vi "簇转换表格.vi"(11 "引用句柄":refnum<vi>) -> (3 "out":string[][](array[string]))   [LabVIEW 2018]
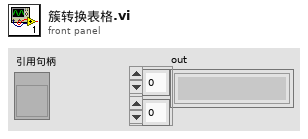
[diagram p1: front panel]
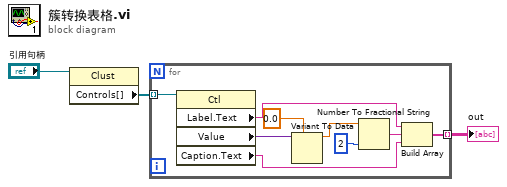
[diagram p0: block diagram]
diagram:
  n1 = property class="Clust"(reference="引用句柄") -> ("Controls[]"=w2:refnum<vi>[])  [unwired: 1 in, 2 out]
  n2 = for {
    tunnel: w2 -> [w10] mode=indexing
    tunnel: [w12] -> w3 mode=indexing
    n3 = property class="Ctl"(reference=w10) -> ("Label.Text"=w11:string, "Value"=w8:variant, "Caption.Text"=w9:string)  [unwired: 1 in, 2 out]
    n4 = Variant To Data(type=0.0, Variant=w8) -> (data=w5:dbl)  [unwired: 1 in, 1 out]
    n5 = Number To Fractional String(number=w5, precision (6)=i16 2 ("精度(6)")) -> (F-format string=w6:string)  [unwired: 2 in]
    n6 = Build Array(w11, w6, w9) -> (w12:string[])
  }
  "out" <- w3
